vi "Sigma0.vi"(1 "a":u32) -> (0 "S0":u32)   [LabVIEW 2019, in "SHA256.lvlib"]
doc: "Calcuates the S0 variable for the compression phase"
uses:
  Downloads/LabVIEW-Bits-master-2/Cryptographic Services/SHA256/SHA256.lvlib
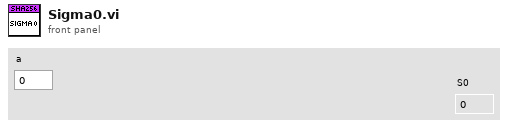
[diagram p1: front panel]
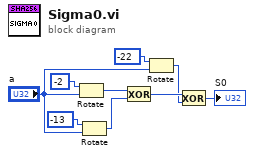
[diagram p0: block diagram]
diagram:
  n1 = Rotate(1:"a", 2:i16 -2 ("y")) -> (0:w5:u32)
  n2 = Rotate(1:"a", 2:i16 -13 ("y")) -> (0:w4:u32)
  n3 = Exclusive Or(1:w4, 2:w5) -> (0:w3:u32)
  n4 = Rotate(1:"a", 2:i16 -22 ("y")) -> (0:w2:u32)
  n5 = Exclusive Or(1:w2, 2:w3) -> (0:→"S0":u32)
